vi "Disconnect.vi"(10 "error in (no error)":errorcluster, 11 "RawSocket Handler in":refnum<class "RawSocket Handler.lvclass">) -> (2 "error out":errorcluster, 3 "RawSocket Handler out":refnum<class "RawSocket Handler.lvclass">)   [LabVIEW 2020, in "wamplv.lvlib" / "RawSocket Handler.lvclass"]
uses:
  RawSocket Handler.lvclass
  RawSocket Handler.lvclass/RawSocket Handler.ctl
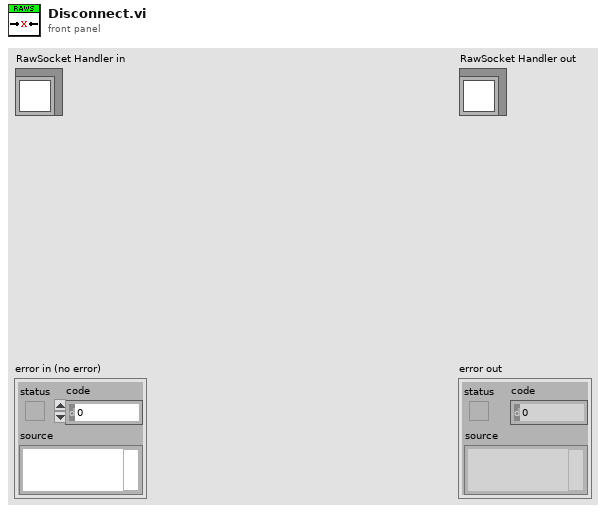
[diagram p1: front panel]
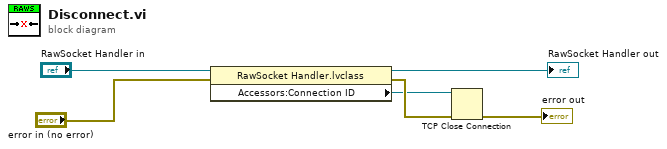
[diagram p0: block diagram]
diagram:
  n1 = property class="RawSocket Handler.lvclass"(reference="RawSocket Handler in", error in="error in (no error)") -> (reference out=→"RawSocket Handler out":refnum<class "RawSocket Handler.lvclass">, error out=w3:errorcluster, "Accessors:Connection ID"=w2:refnum<k5>)
  n2 = TCP Close Connection(connection ID=w2, error in (no error)=w3) -> (error out=→"error out":errorcluster)  [unwired: 1 in, 1 out]
